vi "modify.vi"(8 "error in (no error)":errorcluster, 11 "TrajectoryAK101022Resonance in":refnum<class "TrajectoryAK101022Resonance.lvclass">) -> (0 "error out":errorcluster, 3 "TrajectoryAK101022Resonance out":refnum<class "TrajectoryAK101022Resonance.lvclass">)   [LabVIEW 2010, in "TrajectoryAK101022Resonance.lvclass"]
uses:
  TrajectoryAK101022Resonance.lvclass
  TrajectoryAK101022Resonance.lvclass/TrajectoryAK101022Resonance.ctl
  common/classes/SpaceVector/SpaceVector/SpaceVector.lvclass
panel:
  in  "x scan segment fraction":dbl=0.3 min=0.0 max=1.0 step=0.001
  in  "x offset fly back fraction":dbl=0.1 min=0.0 max=2.0 step=0.001
  in  "x offset fly forward fraction":dbl=0.1 min=0.0 max=2.0 step=0.001
  in  "doneButton":bool
  # "Resonance cycle fraction"
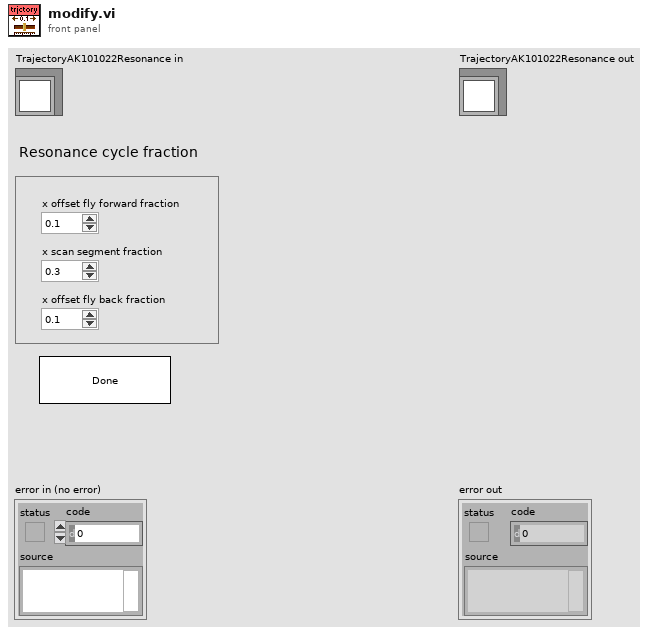
[diagram p1: front panel]
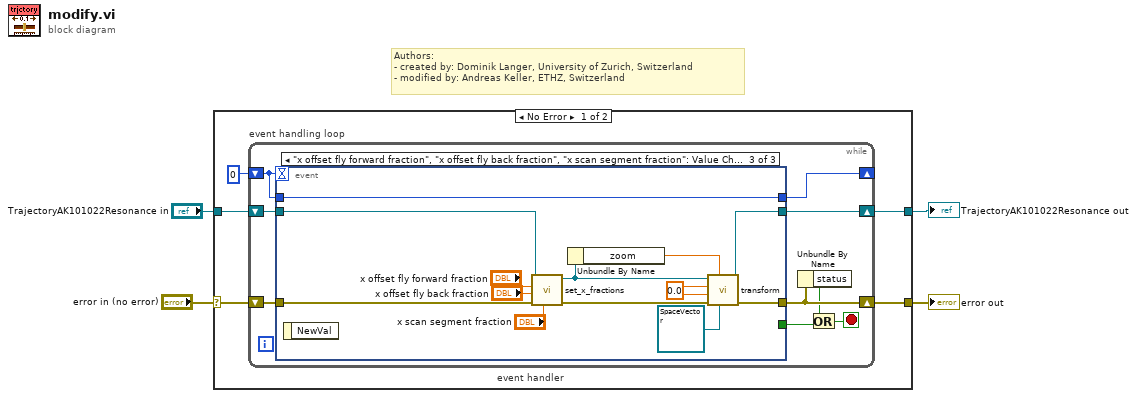
[diagram p0: block diagram]
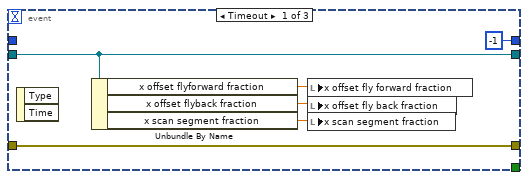
[diagram p2: hidden frame]
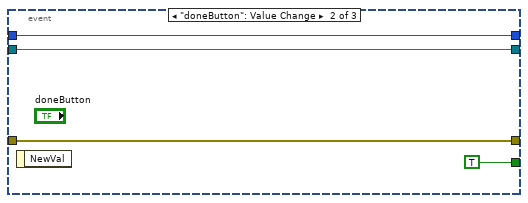
[diagram p3: hidden frame]
diagram:
  # "Authors: \n- created by: Dominik Langer, University of Zurich, Switzerland\n- modified by: Andreas Keller, ETHZ, Switzerland"
  n1 = case shown="No Error" "error in (no error)" {
    selector: "error in (no error)" -> [w9 w43]
    tunnel: [w8 w43] -> w1
    tunnel: "TrajectoryAK101022Resonance in" -> [w7 w42]
    tunnel: [w6 w42] -> w3
    frame No Error {
      n2 = while "event handling loop" {
        shift-right: [w15] -> w8
        shift-left: w9 -> [w18]
        shift-right: [w10] -> _
        shift-left: 0 -> [w11]
        shift-right: [w16] -> w6
        shift-left: w7 -> [w17]
        stop <- w12 stop-if-true
        n3 = event "event handler" shown="[2] \"x offset fly forward fraction\", \"x offset fly back fraction\", \"x scan segment fraction\": Value Change" {
          selector: _ -> [_ _ _]
          dyn-events: _ -> [_ _ _]
          timeout: w11 -> [_ _ _]
          tunnel: w18 -> [w24 w28 w41]
          tunnel: [w24 w28 w38] -> w15
          tunnel: w17 -> [w23 w27 w40]
          tunnel: [w23 w27 w37] -> w16
          tunnel: [_ TRUE _] -> w14
          tunnel: [-1 w25 w32] -> w10
          tunnel: w11 -> [_ w25 w32]
          event Timeout {
            n4 = event-data() -> ()  [unwired: 1 in, 2 out]
            n5 = Unbundle By Name(w23) -> ("x offset flyforward fraction"=w21:dbl, "x offset flyback fraction"=w20:dbl, "x scan segment fraction"=w19:dbl)
            n6 = local write "x offset fly forward fraction"(w21) -> ()
            n7 = local write "x offset fly back fraction"(w20) -> ()
            n8 = local write "x scan segment fraction"(w19) -> ()
          }
          event "doneButton": Value Change {
            n9 = event-data() -> ()  [unwired: 1 in, 1 out]
          }
          event "x offset fly forward fraction", "x offset fly back fraction", "x scan segment fraction": Value Change {
            w33 = dbl[unit] 0.0 ("z angle (phi)")
            n10 = event-data() -> ()  [unwired: 1 in, 1 out]
            n11 = call-dynamic "set_x_fractions.vi"("x scan segment fraction"="x scan segment fraction", "error in (no error)"=w41, "x offset fly back fraction"="x offset fly back fraction", "x offset fly forward fraction"="x offset fly forward fraction", "TrajectoryAK101022Resonance in"=w40) -> ("error out"=w39:errorcluster, "TrajectoryAK101022Resonance out"=w36:refnum<class "TrajectoryAK101022Resonance.lvclass">)  [unwired: 5 in]
            n12 = Unbundle By Name(w36) -> ("zoom"=w35:dbl)
            n13 = call-dynamic "transform.vi"("offset"=refnum<class "SpaceVector.lvclass"> refnum, "zoom"=w35, "error in (no error)"=w39, "x angle (psi)"=w33, "z angle (phi)"=w33, "TrajectoryAK101022Resonance in"=w36) -> ("error out"=w38:errorcluster, "TrajectoryAK101022Resonance out"=w37:refnum<class "TrajectoryAK101022Resonance.lvclass">)  [unwired: 4 in]
          }
        }
        n14 = Unbundle By Name(w15) -> ("status"=w13:bool)
        n15 = Or(x=w13, y=w14) -> (x .or. y?=w12:bool)
      }
    }
    frame Error {
    }
  }
  "error out" <- w1
  "TrajectoryAK101022Resonance out" <- w3
